vi "scouting.vi"() -> ()   [LabVIEW 2017]
panel:
  in  "Average Score":string
  in  "Operation":u16(ring) items=["Input File as Path", "Input File as Refnum", "Specifying a Format String"]
  out "Read Time":timestamp
  out "Read Boolean":bool
  out "Read String":string
  out "Write Time":timestamp
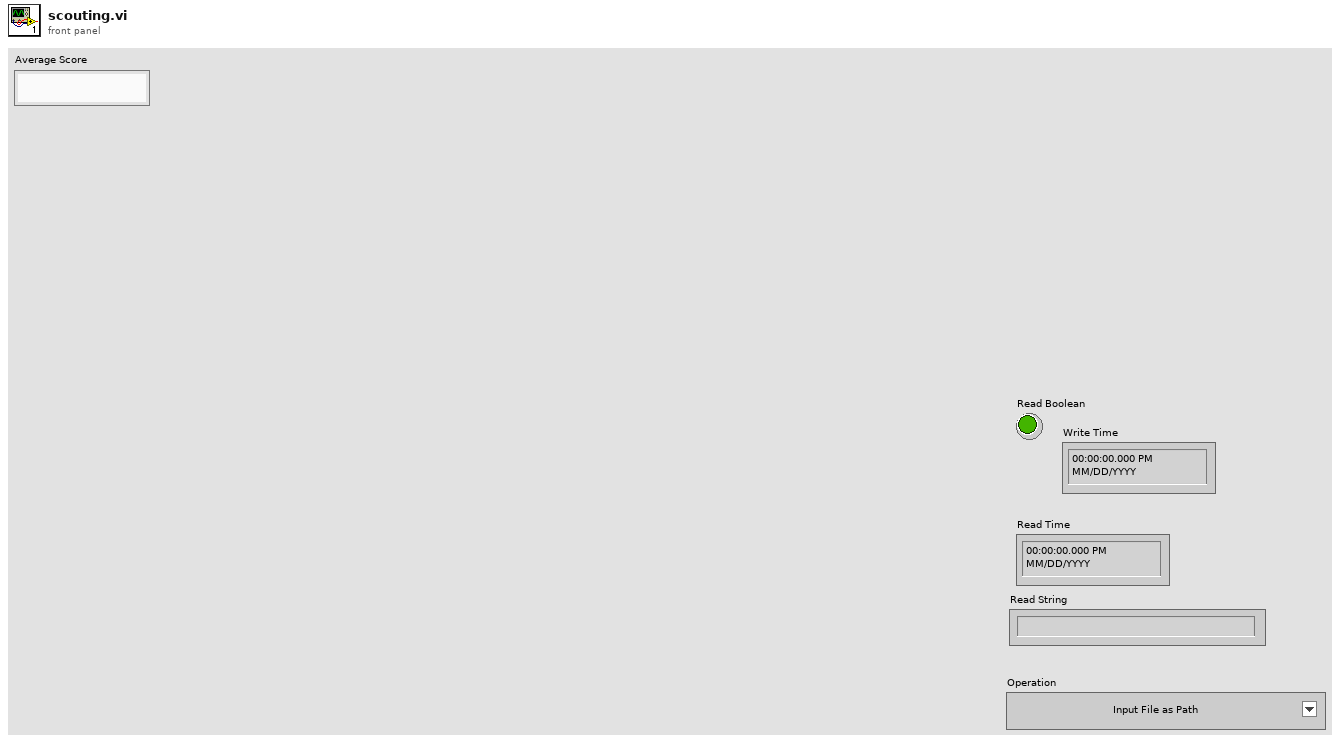
[diagram p1: front panel]
types:
  T1 = enum16{"open", "replace", "create", "open or create", "replace or create", "replace or create with confirmation"}
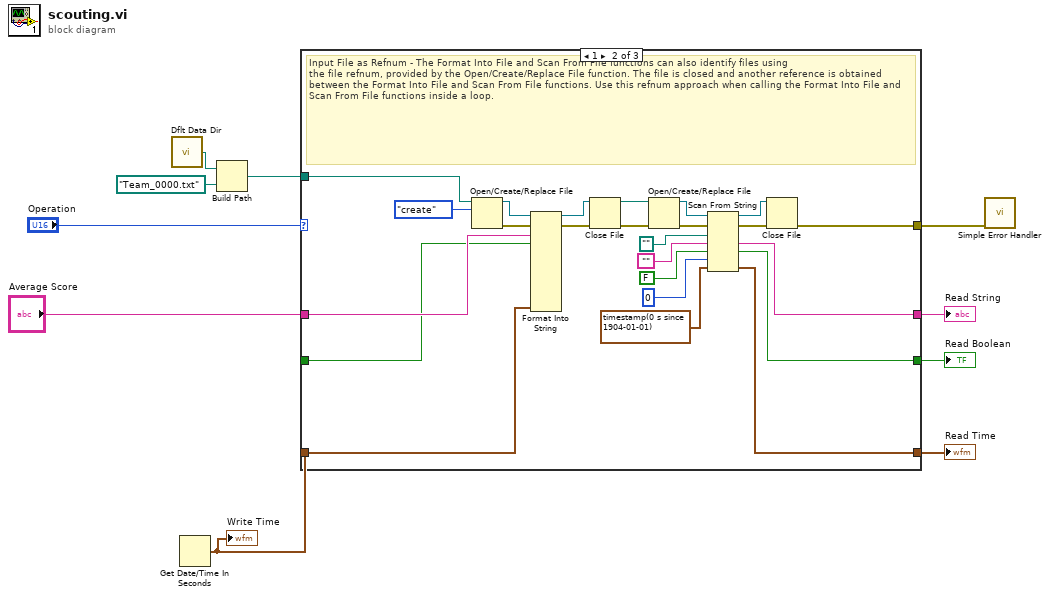
[diagram p0: block diagram]
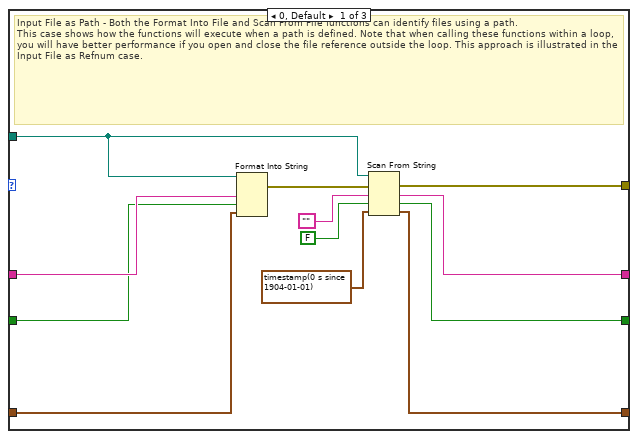
[diagram p2: hidden frame]
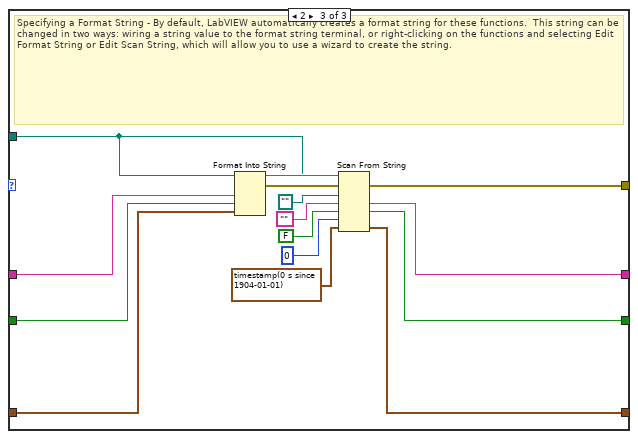
[diagram p3: hidden frame]
diagram:
  n1 = call <vilib>:"Dflt Data Dir.vi"() -> ("App:Default Data Directory"=w4:path)
  n2 = Get Date/Time In Seconds() -> (seconds since 1Jan1904=w10:timestamp)
  "Write Time" <- w10
  n3 = Build Path(base path=w4, name or relative path=path "Team_0000.txt" ("default name")) -> (appended path=w2:path)
  n4 = case shown="1" "Operation" {
    tunnel: [w22 w38 w60] -> w3
    tunnel: "Average Score" -> [w21 w36 w59]
    tunnel: [w20 w35 w58] -> w11
    tunnel: w10 -> [w17 w24 w57]
    tunnel: [w15 w27 w51] -> w9
    tunnel: [w14 w28 w50] -> w8
    tunnel: [w13 w29 w49] -> w7
    tunnel: w2 -> [w12 w26 w48]
    frame 0, Default {
      # "Input File as Path - Both the Format Into File and Scan From File functions can identify files using a path.  \nThis case shows how the functions will execute when a path is defined. Note that when calling these functions within a loop, you will have better performance if you open and close the file reference outside the loop. This approach is illustrated in the Input File as Refnum case."
      n5 = Format Into String(initial string=w12, w21, w20, w17) -> (error out=w23:errorcluster)  [unwired: 2 in, 1 out]
      n6 = Scan From String(w12, w23, default 1="", default 2=FALSE, default 3=timestamp(0 s since 1904-01-01) ("seconds since 1Jan1904")) -> (w22:errorcluster, output 1=w15:string, output 2=w14:bool, output 3=w13:timestamp)  [unwired: 1 in, 1 out]
    }
    frame 1 {
      # "Input File as Refnum - The Format Into File and Scan From File functions can also identify files using \nthe file refnum, provided by the Open/Create/Replace File function. The file is closed and another reference is obtained between the Format Into File and Scan From File functions. Use this refnum approach when calling the Format Into File and Scan From File functions inside a loop."
      n7 = Open/Create/Replace File(file path (use dialog)=w26, operation (0:open)=T1."create") -> (refnum out=w46:refnum<file>, error out=w40:errorcluster)  [unwired: 1 in, 4 out]
      n8 = Format Into String(initial string=w46, error in=w40, w36, w35, w24) -> (resulting string=w45:refnum<file>, error out=w41:errorcluster)  [unwired: 8 in]
      n9 = Close File(refnum=w45, error in=w41) -> (path=w44:path, error out=w43:errorcluster)
      n10 = Open/Create/Replace File(file path (use dialog)=w44, error in=w43) -> (refnum out=w25:refnum<file>, error out=w37:errorcluster)  [unwired: 5 out]
      n11 = Scan From String(w25, w37, default 1=path "", default 2="", default 3=FALSE, default 4=0, default 5=timestamp(0 s since 1904-01-01) ("seconds since 1Jan1904")) -> (w42:refnum<file>, w39:errorcluster, output 2=w27:string, output 3=w28:bool, output 5=w29:timestamp)  [unwired: 1 in, 2 out]
      n12 = Close File(refnum=w42, error in=w39) -> (error out=w38:errorcluster)  [unwired: 1 out]
    }
    frame 2 {
      # "Specifying a Format String - By default, LabVIEW automatically creates a format string for these functions.  This string can be changed in two ways: wiring a string value to the format string terminal, or right-clicking on the functions and selecting Edit Format String or Edit Scan String, which will allow you to use a wizard to create the string."
      n13 = Format Into String(initial string=w48, w59, w58, w57) -> (format string=w62:string, error out=w61:errorcluster)  [unwired: 1 in, 1 out]
      n14 = Scan From String(w62, w48, w61, default 1=path "", default 2="", default 3=FALSE, default 4=0, default 5=timestamp(0 s since 1904-01-01) ("seconds since 1Jan1904")) -> (w60:errorcluster, output 2=w51:string, output 3=w50:bool, output 5=w49:timestamp)  [unwired: 3 out]
    }
  }
  "Read String" <- w9
  "Read Boolean" <- w8
  "Read Time" <- w7
  n15 = call <vilib>:"Simple Error Handler.vi"("error in (no error)"=w3) -> ()  [unwired: 1 in, 8 out]
